vi "CSConnect.constructor.vi"(0 "name":string, 2 "data in":string, 5 "error in (no error)":errorcluster) -> (14 "i ref out":refnum<vi>, 16 "data out":string, 19 "error out":errorcluster)   [LabVIEW 2014, in "CSConnect.lvlib"]
doc: "This is the constructor of a class.\n\nLicense Agreement for this software:\n\nCopyright (C)\nGesellschaft für Schwerionenforschung, GSI\nPlanckstr. 1\n64291 Darmstadt\nGermany\n\nContact: D.Beck@gsi.de \n\nThis program is free software; you can redistribute it and/or modify it under the terms of the \nGNU General Public License as published by the Free Software Foundation; either version 2 of \nthe license, or (at your option) any later version.\n\nThis program is distributed in the hope that it will be useful, but WITHOUT ANY WARRANTY; \nwithout even the implied warranty of MERCHANTABILITY or FITNESS FOR A PARTICULAR PURPOSE. See the GNU General License for more details (http://www.gnu.org).\n\nGesellschaft für Schwerionenforschung, GSI\nPlanckstr. 1, 64291 Darmstadt, Germany\nFor all questions and ideas contact: M.Richter@gsi.de, H.Brand@gsi.de or D.Beck@gsi.de.\nLast update: 16-JUN-2004"
uses:
  CSConnect.lvlib
  CSCore/CSApplicationBaseClasses/DeviceBase/DeviceBase.myEventNames.ctl
  CSCore/CSApplicationBaseClasses/PSChannelBase/PSChannelBase.myEventNames.ctl
  CSConnect.i attribute.ctl
  CSCore/CSSystem/CoreLib/CoreLib.string 2 byte array.vi
  CSCore/CSSystem/CSSystemLib/CSSystemLib.lvlib
  CSCore/CSApplicationBaseClasses/PSChannelBase/PSChannelBase.lvlib
  CSCore/CSApplicationBaseClasses/DeviceBase/DeviceBase.lvlib
  CSCore/BaseProcess/BaseProcess.lvlib
  CSCore/CSObj/CSObj.lvlib
  CSCore/CSSystem/CoreLib/CoreLib.lvlib
  CSlibraries-extern/DimLVEvent/LVDimInterface/LVDimInterface.lvlib
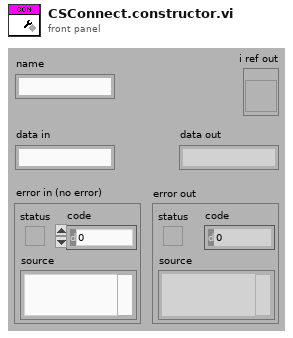
[diagram p1: front panel]
types:
  T1 = typedef "CSConnect.lvlib/CSConnect.i attribute.ctl" = cluster{"In-Array":cluster{"Alias":string, "Value":dbl, "neededOuts":bool[]}[], "Out-Array":cluster{"ObjectName":string, "VoltFunctionName":string, "OnOffFunctionName":string, "Channel":string, "Calculation-Formula":string}[], "OutChannelsID":i32, "InOutMatrixID":i32}
  T2 = enum16{"SetAttribute", "GetAttribute", "CreateAttribute", "DestroyAttribute", "DestroyAllAtributes"}
  T3 = typedef "PSChannelBase.lvlib/PSChannelBase.myEventNames.ctl" = enum16{"lvmsg://EmergencyOff", "lvmsg://SetOnOff", "lvmsg://GetOnOff", "lvmsg://SetVoltage", "lvmsg://GetVoltage", "lvmsg://SetCurrent", "lvmsg://GetCurrent", "lvmsg://SetTripCurrent", "lvmsg://GetTripCurrent", "lvmsg://SetRampUpSpeed", "lvmsg://GetRampUpSpeed", "lvmsg://SetRampDownSpeed", "lvmsg://GetRampDownSpeed", "lvmsg://SetChannelOnOff", "lvmsg://GetChannelOnOff", "lvmsg://SetChannelVoltage", "lvmsg://GetChannelVoltage", "lvmsg://SetChannelCurrent", "lvmsg://GetChannelCurrent", "lvmsg://SetChannelTripCurrent", "lvmsg://GetChannelTripCurrent", "lvmsg://SetChannelRampUpSpeed", "lvmsg://GetChannelRampUpSpeed", "lvmsg://SetChannelRampDownSpeed", "lvmsg://GetChannelRampDownSpeed"}
  T4 = typedef "DeviceBase.lvlib/DeviceBase.myEventNames.ctl" = enum16{"lvmsg://Initialize", "lvmsg://Close", "lvmsg://Configure", "lvmsg://Reset", "lvmsg://IDQuery"}
  T5 = typedef "CSObj.lvlib/CSObj.i attribute.ctl" = cluster{"VI Refnum":refnum<vi>, "Front Panel Ref":refnum<vi>, "semaphore":T6, "date of birth":dbl, "ageID":i32, "systemID":i32, "classID":i32, "conditionID":i32, "DefaultPanelType":u16}
  T6 = typedef "Semaphore RefNum" = refnum<k1>
  T7 = typedef "BaseProcess.lvlib/BaseProcess.i attribute.ctl" = cluster{"EventStatus":string, "EventError":i32, "PresetEvtWatchD":i32, "PresetPdcWatchD":i32, "EventTimeout":i32, "PeriodicInterval":i32, "Interface":string[], "Address":string[], "Special":string[], "PeriodicError":i32, "PeriodicStatus":string, "SuperProc":string, "Descriptors":T8[], "CaseRef":refnum<vi>, "PdcRef":refnum<vi>, "Thread Ref":refnum<vi>, "eventErrorID":i32, "eventStatusID":i32, "periodicErrorID":i32, "periodicStatusID":i32, "pdcCtrID":i32}
  T8 = typedef "BaseProcess.lvlib/BaseProcess.descriptor definition.ctl" = cluster{"selector":string, "descriptor":T9}
  T9 = typedef "BaseProcess.lvlib/BaseProcess.descriptor string definition.ctl" = string
  T10 = cluster{"Interface":string, "Interface":string, "Interface":string, "Interface":string, "String":string}
  T11 = enum16{"simple", "synchronous", "asynchronous", "notification"}
  T12 = typedef "CoreDefs.rawDataType.ctl" = i8[]
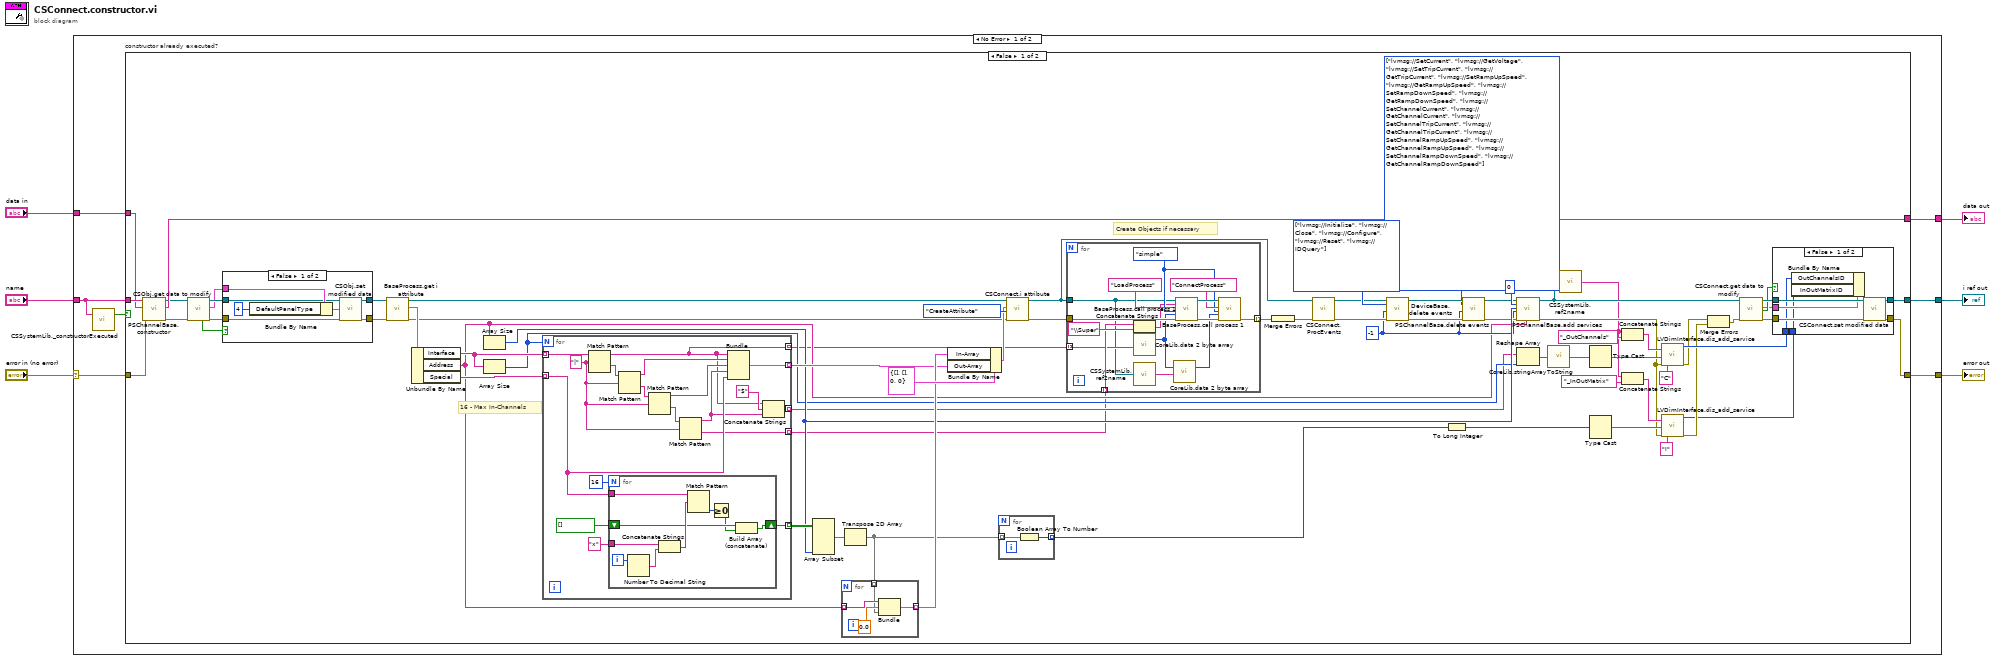
[diagram p0: block diagram]
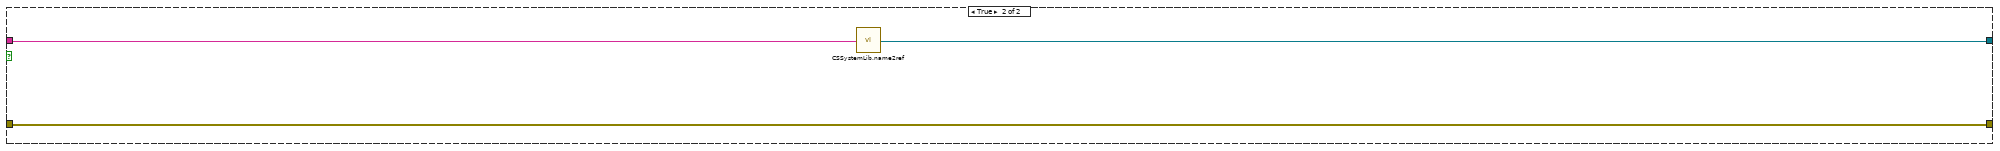
[diagram p4: hidden frame]
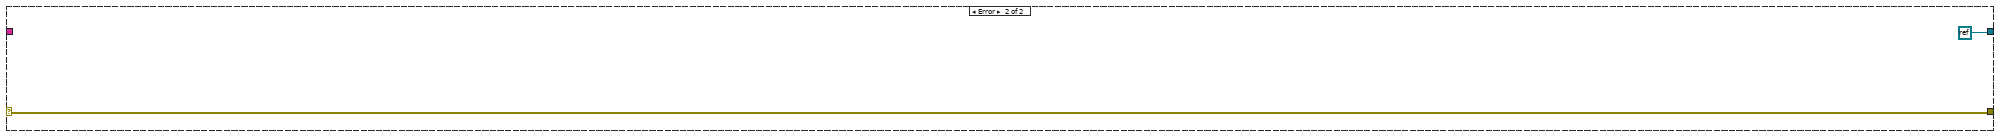
[diagram p5: hidden frame]
diagram:
  n1 = case shown="No Error" "error in (no error)" {
    selector: "error in (no error)" -> [w11 w155]
    tunnel: "name" -> [w10 _]
    tunnel: [w13 refnum<k0> refnum ("Not a Refnum Constant")] -> w5
    tunnel: [w12 w155] -> w4
    tunnel: "data in" -> [w8 _]
    tunnel: [w7 _] -> w1
    frame No Error {
      n2 = call "CSSystemLib._constructorExecuted.vi"("name"=w10) -> ("constructor executed?"=w9:bool)  [unwired: 18 in]
      n3 = case "constructor already executed?" shown="False" w9 {
        tunnel: w10 -> [w83 w154]
        tunnel: [w39 w153] -> w13
        tunnel: [w40 w152] -> w12
        tunnel: w11 -> [w82 w152]
        tunnel: w8 -> [w81 _]
        tunnel: [w74 _] -> w7
        frame False {
          w75 = T3[] [enum."lvmsg://SetCurrent", enum."lvmsg://GetVoltage", enum."lvmsg://SetTripCurrent", enum."lvmsg://GetTripCurrent", enum."lvmsg://SetRampUpSpeed", enum."lvmsg://GetRampUpSpeed", enum."lvmsg://SetRampDownSpeed", enum."lvmsg://GetRampDownSpeed", enum."lvmsg://SetChannelCurrent", enum."lvmsg://GetChannelCurrent", enum."lvmsg://SetChannelTripCurrent", enum."lvmsg://GetChannelTripCurrent", enum."lvmsg://SetChannelRampUpSpeed", enum."lvmsg://GetChannelRampUpSpeed", enum."lvmsg://SetChannelRampDownSpeed", enum."lvmsg://GetChannelRampDownSpeed"] items=["lvmsg://EmergencyOff", "lvmsg://SetOnOff", "lvmsg://GetOnOff", "lvmsg://SetVoltage", "lvmsg://GetVoltage", "lvmsg://SetCurrent", "lvmsg://GetCurrent", "lvmsg://SetTripCurrent", "lvmsg://GetTripCurrent", "lvmsg://SetRampUpSpeed", "lvmsg://GetRampUpSpeed", "lvmsg://SetRampDownSpeed", "lvmsg://GetRampDownSpeed", "lvmsg://SetChannelOnOff", "lvmsg://GetChannelOnOff", "lvmsg://SetChannelVoltage", "lvmsg://GetChannelVoltage", "lvmsg://SetChannelCurrent", "lvmsg://GetChannelCurrent", "lvmsg://SetChannelTripCurrent", "lvmsg://GetChannelTripCurrent", "lvmsg://SetChannelRampUpSpeed", "lvmsg://GetChannelRampUpSpeed", "lvmsg://SetChannelRampDownSpeed", "lvmsg://GetChannelRampDownSpeed"] ("events")
          w80 = T4[] [enum."lvmsg://Initialize", enum."lvmsg://Close", enum."lvmsg://Configure", enum."lvmsg://Reset", enum."lvmsg://IDQuery"] items=["lvmsg://Initialize", "lvmsg://Close", "lvmsg://Configure", "lvmsg://Reset", "lvmsg://IDQuery"] ("events")
          w52 = -1 ("ms timeout (10000)")
          # "Create Objects if necessary"
          # "16 - Max In-Channels"
          n4 = call "PSChannelBase.constructor.vi"("name"=w83, "data in"=w81, "error in (no error)"=w82) -> ("i ref out"=w60:refnum<vi>, "data out"=w74:string, "error out"=w61:errorcluster)  [unwired: 14 in]
          n5 = call "CSObj.get data to modify.vi"("i ref in"=w60, "error in (no error)"=w61) -> ("i ref out"=w64:refnum<vi>, "i attribute"=w62:T5, "timed out"=w65:bool, "error out"=w63:errorcluster)  [unwired: 14 in]
          n6 = case shown="False" w65 {
            tunnel: [w116 w120] -> w59
            tunnel: w64 -> [w117 w120]
            tunnel: [w114 w119] -> w58
            tunnel: w63 -> [w115 w119]
            tunnel: w62 -> [w118 _]
            frame False {
              n7 = Bundle By Name(cluster=w118, "DefaultPanelType"=u16 4) -> (w113:T5)
              n8 = call "CSObj.set modified data.vi"("i ref in"=w117, "i attribute"=w113, "error in (no error)"=w115) -> ("i ref out"=w116:refnum<vi>, "error out"=w114:errorcluster)  [unwired: 15 in]
            }
            frame True {
            }
          }
          n9 = call "BaseProcess.get i attribute.vi"("i ref in"=w59, "error in (no error)"=w58) -> ("i ref out"=w51:refnum<vi>, "i attribute"=w73:T7, "error out"=w50:errorcluster)  [unwired: 15 in]
          n10 = Unbundle By Name(w73) -> ("Interface"=w66:string[], "Address"=w18:string[], "Special"=w72:string[])
          n11 = Array Size(array=w18) -> (size(s)=w55:i32)
          n12 = Array Size(array=w66) -> (size(s)=w49:i32)
          n13 = for {
            N: w49 -> [_]
            tunnel: w66 -> [w142] mode=indexing
            tunnel: w72 -> [w130] mode=indexing
            tunnel: [w141] -> w67 mode=indexing
            tunnel: [w135] -> w56 mode=indexing
            tunnel: [w132] -> w48 mode=indexing
            tunnel: [w126] -> w15 mode=indexing
            tunnel: [w125] -> w14 mode=indexing
            w129 = "|" ("regular expression")
            n14 = Match Pattern(string=w142, regular expression=w129) -> (before substring=w125:string, after substring=w140:string)  [unwired: 1 in, 2 out]
            n15 = for {
              N: 16 -> [_]
              tunnel: w130 -> [w151]
              tunnel: "x" ("string") -> [w149]
              shift-right: [w143] -> w135
              shift-left: bool[] [] -> [w145]
              i -> [w150]
              n16 = Number To Decimal String(number=w150) -> (decimal integer string=w148:string)  [unwired: 1 in]
              n17 = Concatenate Strings(w149, w148) -> (w147:string)
              n18 = Match Pattern(string=w151, regular expression=w147) -> (offset past match=w146:i32)  [unwired: 1 in, 3 out]
              n19 = Greater Or Equal To 0?(x=w146) -> (x >= 0?=w144:bool)
              n20 = Build Array (concatenate)(w145, w144) -> (w143:bool[])
            }
            n21 = Match Pattern(string=w140, regular expression=w129) -> (before substring=w139:string, after substring=w134:string)  [unwired: 1 in, 2 out]
            n22 = Match Pattern(string=w134, regular expression=w129) -> (before substring=w133:string, after substring=w128:string)  [unwired: 1 in, 2 out]
            n23 = Match Pattern(string=w128, regular expression=w129) -> (before substring=w127:string, after substring=w126:string)  [unwired: 1 in, 2 out]
            n24 = Bundle("Interface"=w125, "Interface"=w139, "Interface"=w133, "Interface"=w127, "String"=w130) -> (w141:T10)  [unwired: 1 in]
            n25 = Concatenate Strings(w125, "$", w127) -> (w132:string)
          }
          n26 = Array Subset(array=w56, length (col)=w55) -> (w57:bool[][])  [unwired: 3 in]
          n27 = Transpose 2D Array(2D array=w57) -> (transposed array=w32:bool[][])
          n28 = for {
            tunnel: w18 -> [w123] mode=indexing
            tunnel: [w122] -> w68 mode=indexing
            tunnel: w32 -> [w121] mode=indexing
            n29 = Bundle("String"=w123, 0.0, w121) -> (w122:cluster{"String":string, dbl, bool[]})  [unwired: 1 in]
          }
          n30 = Bundle By Name(cluster=T1 {"In-Array"=[], "Out-Array"=[], "OutChannelsID"=0, "InOutMatrixID"=0} ("CLASS.i attribute"), "In-Array"=w68, "Out-Array"=w67) -> (w70:T1)
          n31 = for {
            tunnel: w32 -> [w101] mode=indexing
            tunnel: [w100] -> w23 mode=indexing
            n32 = Boolean Array To Number(Boolean array=w101) -> (number=w100:u32)
          }
          n33 = call "CSConnect.i attribute.vi"("VI Refnum"=w51, "CLASS.i attribute"=w70, "Action"=T2."CreateAttribute", "error in (no error)"=w50) -> ("VI Refnum out"=w16:refnum<vi>, "error out"=w20:errorcluster)  [unwired: 13 in, 1 out]
          n34 = for {
            tunnel: w16 -> [w85]
            tunnel: w20 -> [w97]
            tunnel: [w95] -> w19 mode=indexing
            tunnel: w15 -> [w89] mode=indexing
            tunnel: w14 -> [w88] mode=indexing
            w92 = T11."simple" ("CallType")
            n35 = Concatenate Strings(w89, "\\Super" ("string")) -> (w90:string)
            n36 = call-poly "CoreLib.data 2 byte array.vi"("string"=w88) -> ("byteArray out"=w87:T12)  [unwired: 18 in]
            n37 = call "CSSystemLib.ref2name.vi"("obj refnum"=w85) -> ("name"=w86:string)
            n38 = call-poly "CoreLib.data 2 byte array.vi"("byteArray"=w87, "string"=w86) -> ("byteArray out"=w91:T12)  [unwired: 17 in]
            n39 = call "BaseProcess.call process 1.vi"("i ref in"=w85, "Object"=w90, "Selector"="LoadProcess", "CallType"=w92, "Data"=w87, "error in (no error)"=w97) -> ("i ref out"=w98:refnum<vi>, "error out"=w96:errorcluster)  [unwired: 11 in, 1 out]
            n40 = call "BaseProcess.call process 1.vi"("i ref in"=w98, "Selector"="ConnectProcess", "CallType"=w92, "Data"=w91, "error in (no error)"=w96) -> ("error out"=w95:errorcluster)  [unwired: 12 in, 2 out]
          }
          n41 = Merge Errors(w19) -> (w17:errorcluster)
          n42 = call "CSConnect.ProcEvents.vi"("i ref in"=w16, "error in (no error)"=w17) -> ("i ref out"=w79:refnum<vi>, "error out"=w78:errorcluster)  [unwired: 16 in]
          n43 = call "DeviceBase.delete events.vi"("i ref in"=w79, "events"=w80, "ms timeout (10000)"=w52, "error in (no error)"=w78) -> ("i ref out"=w77:refnum<vi>, "error out"=w76:errorcluster)  [unwired: 13 in, 1 out]
          n44 = To Long Integer(number=w23) -> (32bit integer=w22:i32[])
          n45 = call "PSChannelBase.delete events.vi"("i ref in"=w77, "events"=w75, "ms timeout (10000)"=w52, "error in (no error)"=w76) -> ("i ref out"=w53:refnum<vi>, "error out"=w54:errorcluster)  [unwired: 13 in, 1 out]
          n46 = call "PSChannelBase.add services.vi"("i ref in"=w53, "defaultChannelIndex"=0, "nofChannels"=w55, "ms timeout (10000)"=w52, "error in (no error)"=w54, "logicalNames"=w18) -> ("i ref out"=w41:refnum<vi>, "error out"=w27:errorcluster)  [unwired: 11 in, 1 out]
          n47 = Reshape Array(w48, w49) -> (w47:string[])
          n48 = call "CoreLib.stringArrayToString.vi"("Array"=w47) -> ("String"=w46:string)
          n49 = call "CSSystemLib.ref2name.vi"("obj refnum"=w41) -> ("name"=w21:string)
          n50 = Type Cast(x=w46) -> (*(type *) &x=w44:string)  [unwired: 1 in]
          n51 = Type Cast(x=w22) -> (*(type *) &x=w30:string)  [unwired: 1 in]
          n52 = Concatenate Strings(w21, "_OutChannels" ("string")) -> (w43:string)
          n53 = Concatenate Strings(w21, "_InOutMatrix" ("string")) -> (w29:string)
          n54 = call "LVDimInterface.dis_add_service.vi"("serviceName"=w43, "typeDescriptor"="C", "data"=w44, "error in (no error)"=w27) -> ("my_serviceID"=w34:i32, "error out"=w33:errorcluster)  [unwired: 14 in]
          n55 = call "LVDimInterface.dis_add_service.vi"("serviceName"=w29, "typeDescriptor"="I", "data"=w30, "error in (no error)"=w27) -> ("my_serviceID"=w24:i32, "error out"=w25:errorcluster)  [unwired: 14 in]
          n56 = Merge Errors(w33, w25) -> (w26:errorcluster)
          n57 = call "CSConnect.get data to modify.vi"("i ref in"=w41, "error in (no error)"=w26) -> ("i ref out"=w38:refnum<vi>, "i attribute"=w35:T1, "timed out"=w36:bool, "error out"=w37:errorcluster)  [unwired: 14 in]
          n58 = case shown="False" w36 {
            tunnel: [w109 w110] -> w40
            tunnel: [w108 w111] -> w39
            tunnel: w38 -> [w107 w111]
            tunnel: w37 -> [w106 w110]
            tunnel: w35 -> [w105 _]
            tunnel: w34 -> [w103 _]
            tunnel: w24 -> [w102 _]
            frame False {
              n59 = Bundle By Name(cluster=w105, "OutChannelsID"=w103, "InOutMatrixID"=w102) -> (w104:T1)
              n60 = call "CSConnect.set modified data.vi"("i ref in"=w107, "i attribute"=w104, "error in (no error)"=w106) -> ("i ref out"=w108:refnum<vi>, "error out"=w109:errorcluster)  [unwired: 15 in]
            }
            frame True {
            }
          }
        }
        frame True {
          n61 = call "CSSystemLib.name2ref.vi"("name"=w154) -> ("obj refnum"=w153:refnum<vi>)
        }
      }
    }
    frame Error {
    }
  }
  "i ref out" <- w5
  "error out" <- w4
  "data out" <- w1
